vi "ex_CopyPropertiesToUSI.vi"(4 "error in (no error)":errorcluster, 6 "Properties":T1[](array[typedef]), 7 "dup storage refnum":refnum<k20>) -> (0 "error out":errorcluster, 3 "dup storage refnum":refnum<k20>)   [LabVIEW 2020]
uses:
  <vilib>/express/express shared/ExFile.llb/ex_TdmProperty.ctl
  <vilib>/express/express shared/ex_EditUserDefinedProperties/usiDataType.ctl
  <vilib>/Platform/storage/Storage.llb/Set Property (I32).vi
  <vilib>/Platform/storage/Storage.llb/Set Property (DBL).vi
  <vilib>/Platform/storage/Storage.llb/Set Property (String).vi
  <vilib>/Platform/storage/Storage.llb/Set Property (Time Stamp).vi
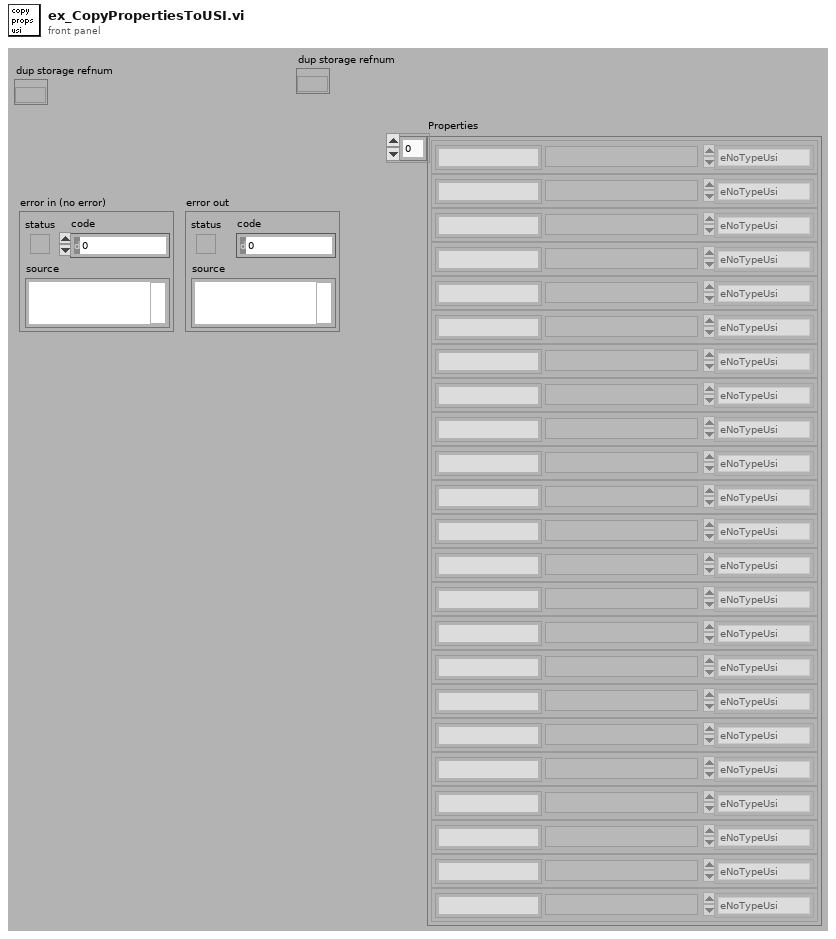
[diagram p1: front panel]
types:
  T1 = typedef "ex_TdmProperty.ctl" = cluster{"Name":string, "Type":T2, "Value":variant}
  T2 = typedef "usiDataType.ctl" = enum16{"eNoTypeUsi", "eInt8Usi", "eInt16Usi", "eInt32Usi", "eInt64Usi", "eUInt8Usi", "eUInt16Usi", "eUInt32Usi", "eUInt64Usi", "eFloat32Usi", "eFloat64Usi", "- 0", "- 1", "- 2", "- 3", "- 4", "- 5", "- 6", "- 7", "- 8", "- 9", "eString8Usi", "eString16Usi", "eStringUsi", "eEnumUsi", "- 10", "- 11", "- 12", "- 13", "- 14", "eTimeUsi", "- 15", "- 16", "- 17", "- 18", "- 19", "- 20", "- 21", "- 22", "- 23", "eInstanceUsi", "eStoreUsi"}
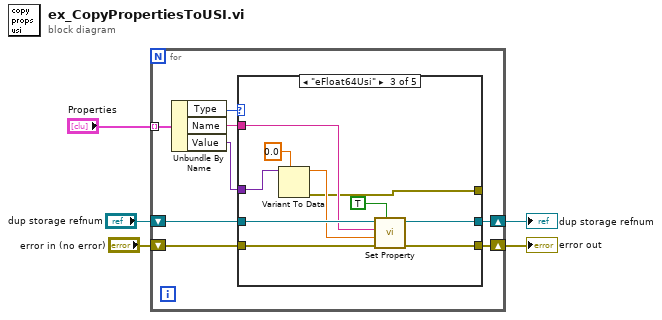
[diagram p0: block diagram]
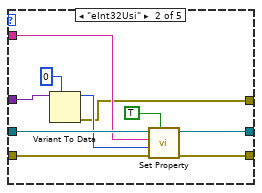
[diagram p3: hidden frame]
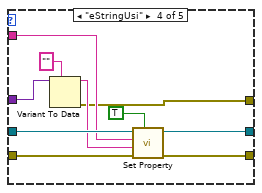
[diagram p4: hidden frame]
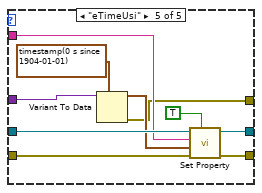
[diagram p5: hidden frame]
diagram:
  n1 = for {
    tunnel: "Properties" -> [w6] mode=indexing
    shift-right: [w7] -> w2
    shift-left: "dup storage refnum" -> [w10]
    shift-right: [w13] -> w5
    shift-left: "error in (no error)" -> [w9]
    n2 = Unbundle By Name(w6) -> ("Type"=w8:T2, "Name"=w11:string, "Value"=w12:variant)
    n3 = case shown="\"eFloat64Usi\"" w8 {
      tunnel: w9 -> [w15 w25 w35 w45 w55]
      tunnel: w10 -> [w14 w23 w33 w43 w53]
      tunnel: [w15 w22 w32 w42 w52] -> w13
      tunnel: w11 -> [_ w18 w31 w41 w51]
      tunnel: w12 -> [_ w21 w30 w40 w50]
      tunnel: [w14 w17 w27 w37 w47] -> w7
      tunnel: [_ w16 w26 w36 w46] -> _
      frame "eNoTypeUsi", Default {
      }
      frame "eInt32Usi" {
        n4 = Variant To Data(type=0, Variant=w21) -> (data=w19:i32, error out=w16:errorcluster)  [unwired: 1 in]
        n5 = call-poly <vilib>:"Set Property.vi"("Create if not found (no:F)"=TRUE, "error in (no error)"=w25, "Value"=w19, "Property name"=w18, "storage refnum"=w23) -> ("error out"=w22:errorcluster, "storage refnum out"=w17:refnum<k20>)  [unwired: 5 out]
      }
      frame "eFloat64Usi" {
        n6 = Variant To Data(type=0.0, Variant=w30) -> (data=w28:dbl, error out=w26:errorcluster)  [unwired: 1 in]
        n7 = call-poly <vilib>:"Set Property.vi"("Create if not found (no:F)"=TRUE, "error in (no error)"=w35, "Value"=w28, "Property name"=w31, "storage refnum"=w33) -> ("error out"=w32:errorcluster, "storage refnum out"=w27:refnum<k20>)  [unwired: 5 out]
      }
      frame "eStringUsi" {
        n8 = Variant To Data(type="", Variant=w40) -> (data=w38:string, error out=w36:errorcluster)  [unwired: 1 in]
        n9 = call-poly <vilib>:"Set Property.vi"("Create if not found (no:F)"=TRUE, "error in (no error)"=w45, "Value"=w38, "Property name"=w41, "storage refnum"=w43) -> ("error out"=w42:errorcluster, "storage refnum out"=w37:refnum<k20>)  [unwired: 5 out]
      }
      frame "eTimeUsi" {
        n10 = Variant To Data(type=timestamp(0 s since 1904-01-01), Variant=w50) -> (data=w49:timestamp, error out=w46:errorcluster)  [unwired: 1 in]
        n11 = call-poly <vilib>:"Set Property.vi"("Create if not found (no:F)"=TRUE, "error in (no error)"=w55, "Value"=w49, "Property name"=w51, "storage refnum"=w53) -> ("error out"=w52:errorcluster, "storage refnum out"=w47:refnum<k20>)  [unwired: 5 out]
      }
    }
  }
  "error out" <- w5
  "dup storage refnum" <- w2
